vi "Final Project GUI with IMU.vi"() -> ()   [LabVIEW 2021]
doc: "This example performs writes and reads on a serial port, as directed by the user. You can press the Write and Read buttons, and change the Read Count, while the example is running.\n\nThe parameters set for the serial port must match the parameters of the connected instrument or device. In this example, the Read Count parameter specifies the number of bytes that the serial port reads. If there were more bytes at the port than the specified number, those bytes would not be read. If there were less bytes at the port than the specified number, you would receive a timeout error.\n\nThis example expands upon the flow control options for XON and XOFF, allowing the user to choose those control characters. Also, the user can enable or disable a termination character. Some devices require a termination character in order to identify the end of command strings. Some devices send a termination character to signify the end of data to be read. This example shows how you can end the Read operation once a termination character is detected in the buffer and/or append a termination character at the end of the Write data."
uses:
  Serial - Settings.ctl
  Serial - XON-XOFF Characters.ctl
  Serial - ASCII Characters-1.ctl
  <vilib>/Instr/_visa.llb/VISA Configure Serial Port (Instr).vi
  <vilib>/picture/picture.llb/Draw True-Color Pixmap.vi
panel:
  out "x*y":dbl
  out "front angle calcs":dbl
  out "ticks":dbl
  out "ResBack":dbl
  out "ResFront":dbl
  out "side angle calcs":dbl
  in  "milliseconds to wait":u32=17
  out "old pwm modifier":dbl
  in  "PWM actuator modifier":dbl
  out "Time used":dbl
  in  "Tab Control":T1(tab)
  in  "Write":bool
  out "Response":string
  in  "Command":string="\n\n"
  in  "Stop":bool
  in  "VISA resource name":refnum<visa-resource-name>="COM7"
  in  "Serial Settings":T2={"baud rate"=115200, "data bits"=8, "parity"=enum."None", "stop bits"=10, "flow control"=0} {"flow control" items=["None"=0, "XON/XOFF"=1, "RTS/CTS"=2, "DTR/DSR"=4]; "stop bits" items=["1.0"=10, "1.5"=15, "2.0"=20]; "data bits" min=5 max=8 step=1; "baud rate" items=["75"=75, "110"=110, "134"=134, "150"=150, "300"=300, "600"=600, "1200"=1200, "1800"=1800, "2400"=2400, "4800"=4800, "7200"=7200, "9600"=9600, "14400"=14400, "19200"=19200, "28800"=28800, "38400"=38400, "56000"=56000, "57600"=57600, "115200"=115200, "128000"=128000, "230400"=230400]}
  in  "End Read on Termination Character?":bool=TRUE
  in  "XON/XOFF Characters":T3={"XON"=enum."DC1", "XOFF"=enum."DC3"}
  in  "End Write on Termination Character?":bool=TRUE
  in  "Termination Character":u8=13 format="%.0x"
  out "Front View":picture
  out "Side View":picture
  out "Front View graph":dbl[](graph)
  out "Side Graph":dbl[](graph)
  in  "stop":bool
  out "IMU angle from PSOC":dbl
  in  "Reset Actuators to 2":bool
  in  "Reset Actuators to Zero":bool
  out "Actuator 1 Length (inches)":string
  out "Actuator 2 Length (inches)":string
  out "Actuator 3 Length (inches)":string
  out "Actuator 4 Length (inches)":string
  out "Actuator 1":dbl[](graph)
  out "Actuator 2":dbl[](graph)
  out "Actuator 3":dbl[](graph)
  out "Actuator 4":dbl[](graph)
  out "Actuator 1\nLength":dbl(slide) scale=0.0..2.0
  out "Actuator 2\nLength":dbl(slide) scale=0.0..2.0
  out "Actuator 3\nLength":dbl(slide) scale=0.0..2.0
  out "Actuator 4\nLength":dbl(slide) scale=0.0..2.0
  out "read buffer":string
  # "TEMPORARY DEBUGGING TOOLS"
  # "Hello! Welcome to the ME and the Boys ME135 Project!\n\nWe designed a mobile self-balancing platform with an actuator on each end. The rover will \nautomatically detect if the platform is not flat, and adjust the actuators accordingly while \ndriving over bumps and rough terrain.\n\nExplanation of each GUI tab:\nSetup - Serial Communication Setup (Change COM port here)\nOrientation Viewer - Plot of pitch and roll angle during operation \nActuator Lengths  - Plot of actuator lengths at each corner"
  # "Serial Communciation Setup Panel"
  # "Instructions:\n1. Using Windows Device Manager take note of the COM port given by Windows to your microcontroller connection\n2. Change the VISA resource name to your COM port from step 1\n3. Run the VI.\n4. Press reset on your microcontroller\n5. The corresponding response should appear in the Response Window\n6. Click Stop to stop the VI."
  # "0xA is equivalent to a '\\n' character, which is a line feed."
  # "Orientation\nViewer"
  # "Actuator Length Overview"
  # "CAR"
  # "car"
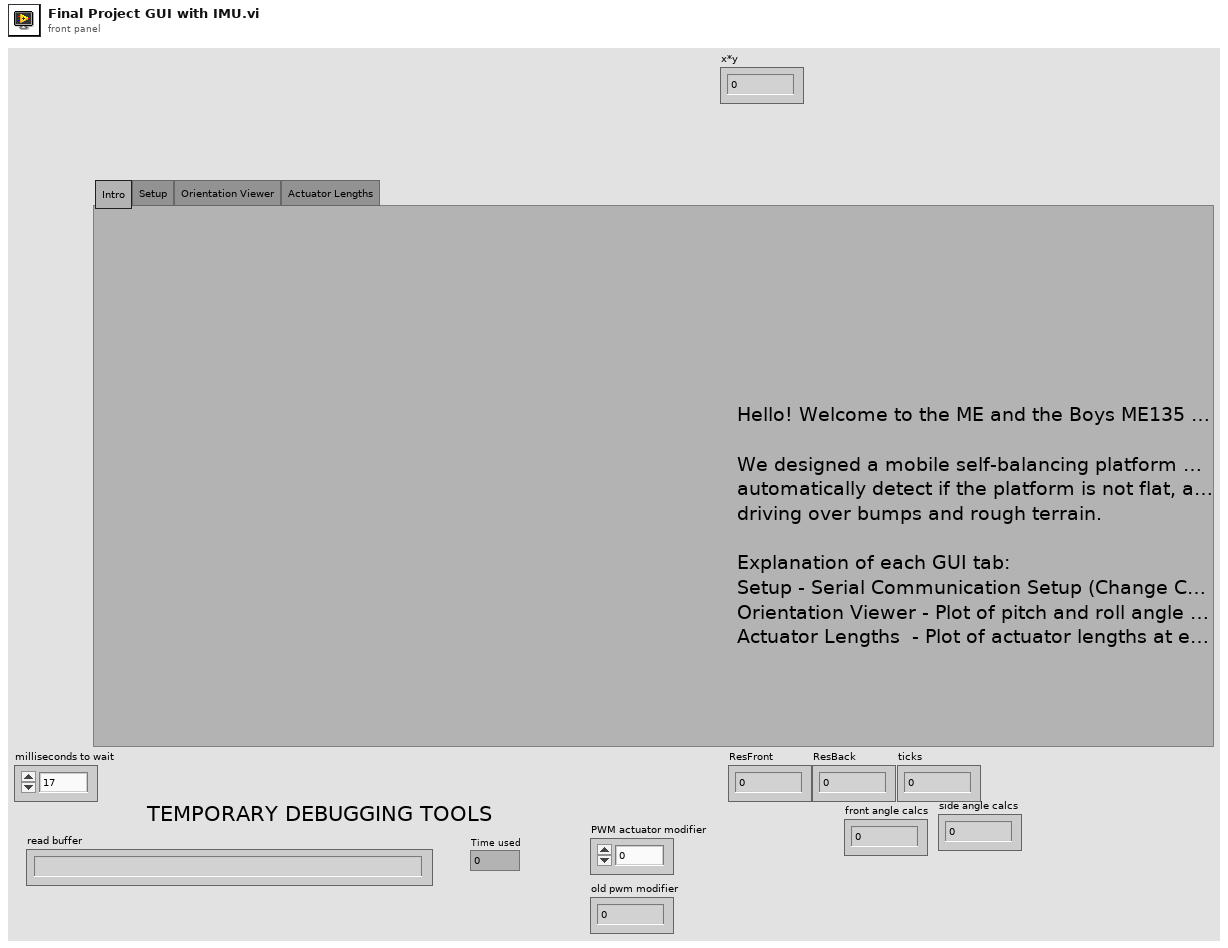
[diagram p1: front panel]
types:
  T1 = enum32{"Intro", "Setup", "Orientation Viewer", "Actuator Lengths"}
  T2 = typedef "Serial - Settings.ctl" = cluster{"baud rate":u32, "data bits":u16, "parity":enum16{"None", "Odd", "Even", "Mark", "Space"}, "stop bits":u16, "flow control":u16}
  T3 = typedef "Serial - XON-XOFF Characters.ctl" = cluster{"XON":T4, "XOFF":T4}
  T4 = typedef "Serial - ASCII Characters-1.ctl" = enum16{"NUL", "SOH", "STX", "ETX", "EOT", "ENQ", "ACK", "BEL", "BS", "HT", "LF", "VT", "FF", "CR", "SO", "SI", "DLE", "DC1", "DC2", "DC3", "DC4", "NAK", "SYN", "ETB", "CAN", "EM", "SUB", "ESC", "FS", "GS", "RS", "US", "SP", "!", "\"", "#", "$", "%", "&", "'", "(", ")", "*", "+", ",", "- (-)", ".", "/", "0", "1", "2", "3", "4", "5", "6", "7", "8", "9", ":", ";", "<", "=", ">", "?", "@", "A", "B", "C", "D", "E", "F", "G", "H", "I", "J", "K", "L", "M", "N", "O", "P", "Q", "R", "S", "T", "U", "V", "W", "X", "Y", "Z", "[", "\\", "]", "^", "_", "`", "a", "b", "c", "d", "e", "f", "g", "h", "i", "j", "k", "l", "m", "n", "o", "p", "q", "r", "s", "t", "u", "v", "w", "x", "y", "z", "{", "|", "}", "~"}
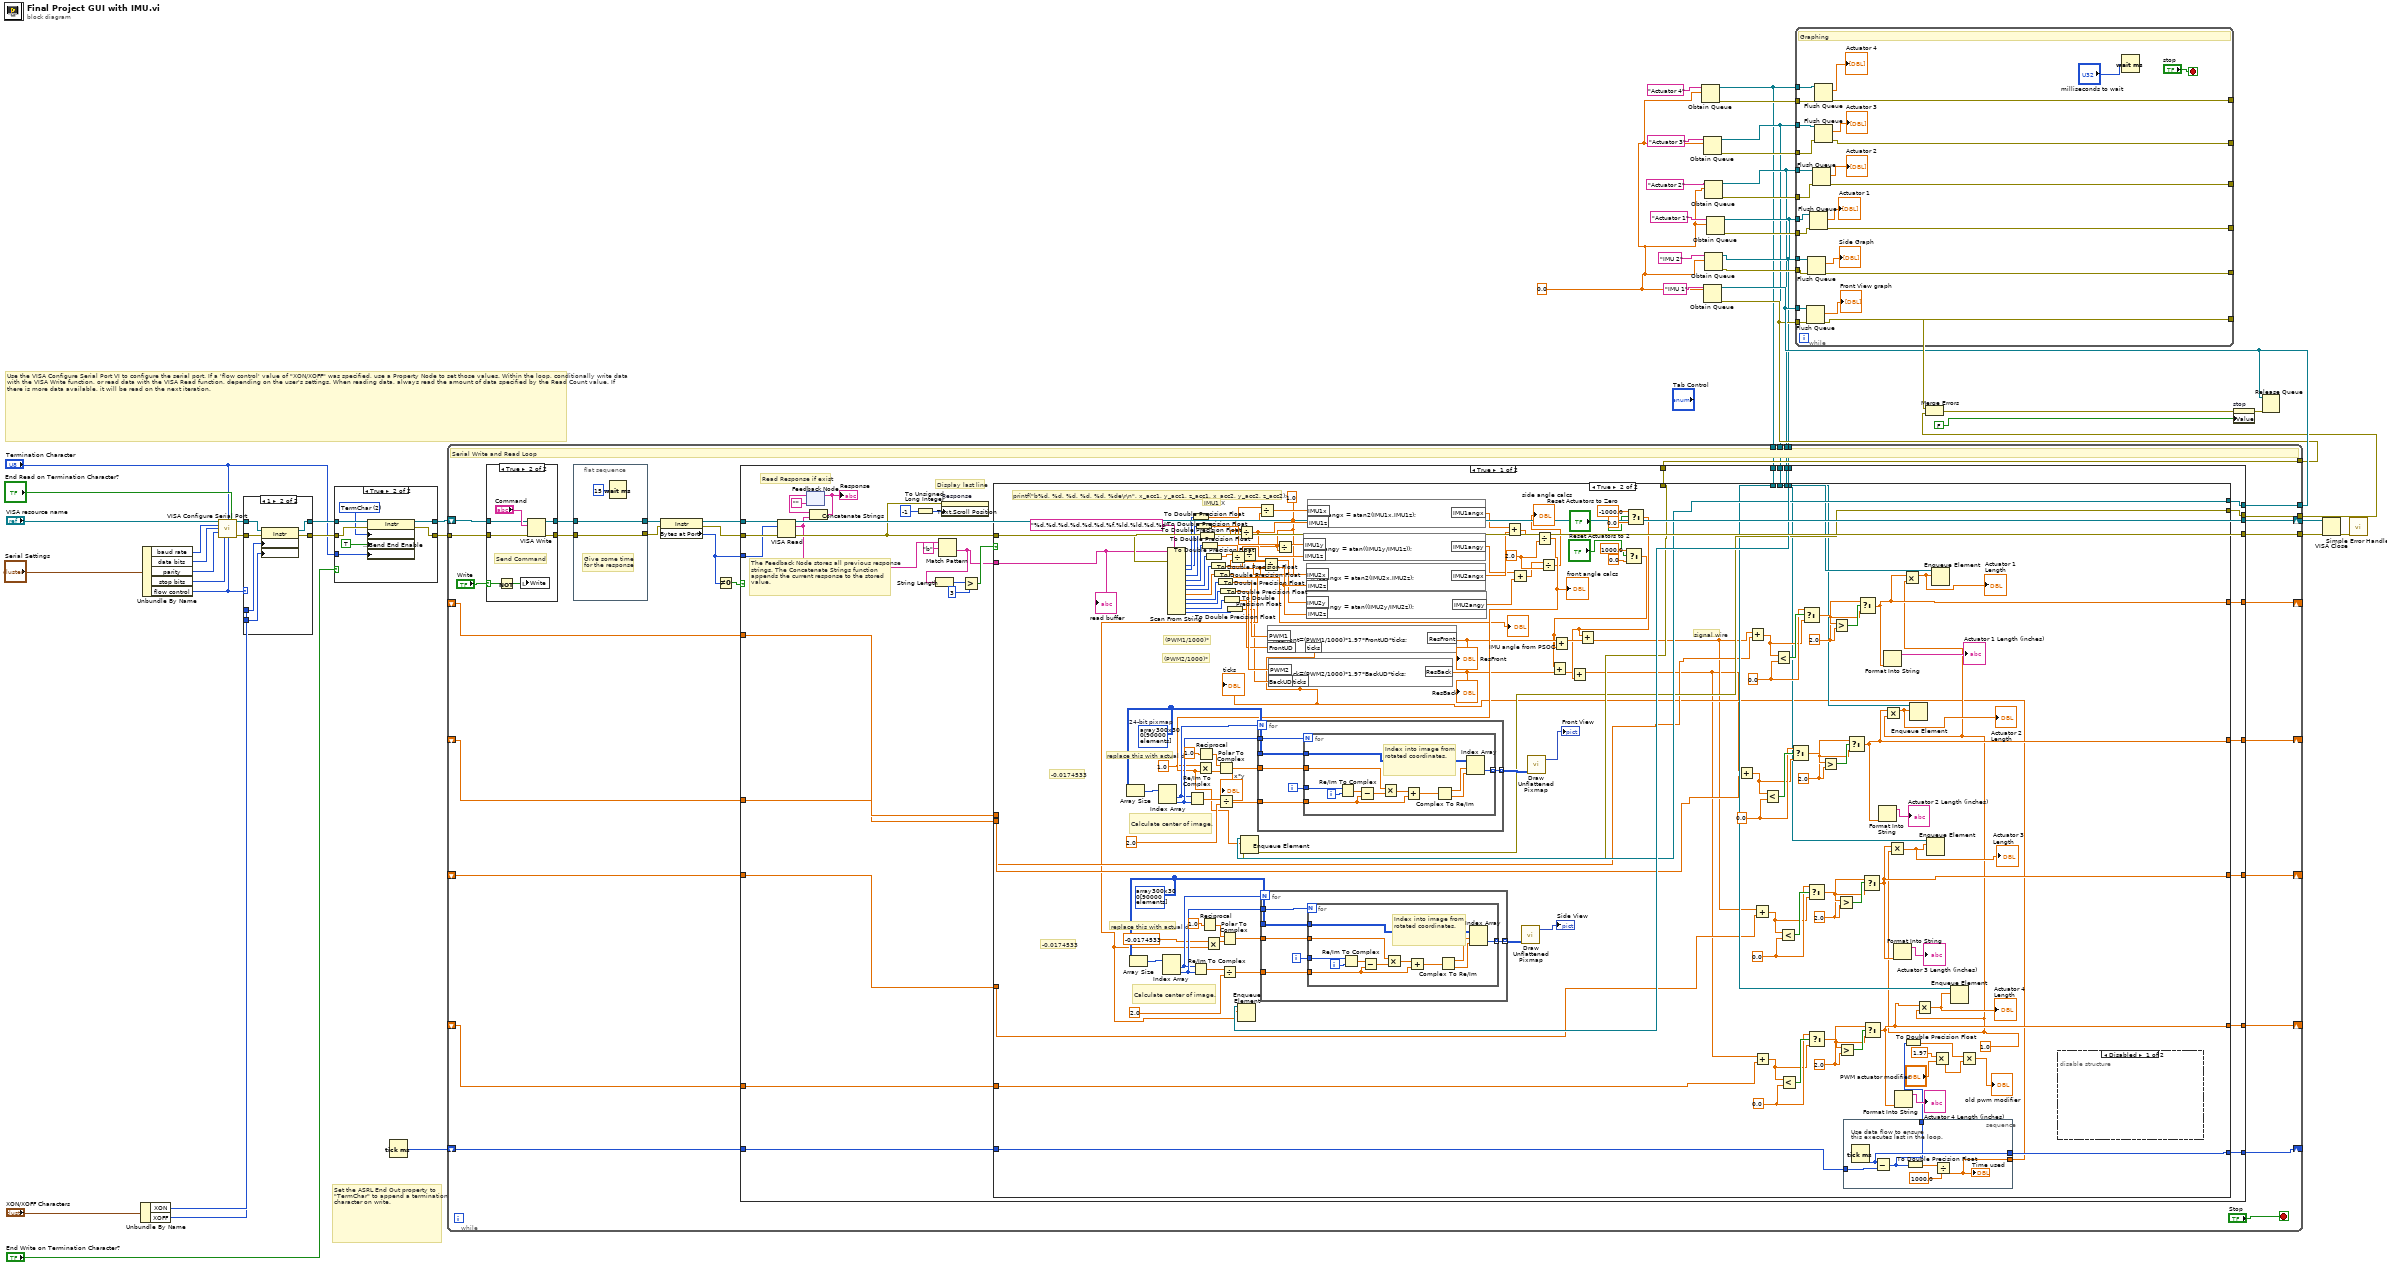
[diagram p0: block diagram]
diagram:
  w2 = 0.0
  # "Set the ASRL End Out property to \"TermChar\" to append a termination character on write."
  # "Use the VISA Configure Serial Port VI to configure the serial port. If a 'flow control' value of \"XON/XOFF\" was specified, use a Property Node to set those values. Within the loop, conditionally write data with the VISA Write function, or read data with the VISA Read function, depending on the user's settings. When reading data, always read the amount of data specified by the Read Count value. If there is more data available, it will be read on the next iteration."
  n1 = Unbundle By Name("XON/XOFF Characters") -> ("XON"=w33:T4, "XOFF"=w32:T4)
  n2 = Unbundle By Name("Serial Settings") -> ("baud rate"=w40:u32, "data bits"=w41:u16, "parity"=w42:enum16{"None", "Odd", "Even", "Mark", "Space"}, "stop bits"=w43:u16, "flow control"=w34:u16)
  n3 = call-poly "VISA Configure Serial Port"("VISA resource name"="VISA resource name", "termination char\n(0xA = '\\n' = LF)"="Termination Character", "Enable Termination\nChar (T)"="End Read on Termination Character?", "baud rate (9600)"=w40, "data bits (8)"=w41, "parity (0:none)"=w42, "stop bits (10: 1 bit)"=w43, "flow control (0:none)"=w34) -> ("VISA resource name out"=w44:refnum<visa-resource-name>, "error out"=w45:errorcluster)  [unwired: 2 in, 4 out]
  n4 = case shown="1" w34 {
    tunnel: [w48 w55] -> w31
    tunnel: [w49 w54] -> w29
    tunnel: w45 -> [w48 w53]
    tunnel: w44 -> [w49 w52]
    tunnel: w33 -> [_ w51]
    tunnel: w32 -> [_ w50]
    frame Default {
    }
    frame 1 {
      n5 = property class="Instr"(reference=w52, error in=w53, "Serial Settings:Flow Control XON Character"=w51, "Serial Settings:Flow Control XOFF Character"=w50) -> (reference out=w54:refnum<visa-resource-name>, error out=w55:errorcluster)
    }
  }
  n6 = case shown="True" "End Write on Termination Character?" {
    tunnel: w29 -> [w56 w64]
    tunnel: w31 -> [w57 w63]
    tunnel: [w56 w62] -> w28
    tunnel: [w57 w61] -> w30
    tunnel: "Termination Character" -> [_ w59]
    frame False {
    }
    frame True {
      w60 = u16 2 items=["None", "LastBit", "TermChar", "Break"] ("Serial Settings:Serial End Mode for Writes")
      n7 = property class="Instr"(reference=w64, error in=w63, "Serial Settings:End Mode for Writes"=w60, "Message Based Settings:Send End Enable"=TRUE, "Message Based Settings:Termination Character"=w59) -> (reference out=w62:refnum<visa-resource-name>, error out=w61:errorcluster)
    }
  }
  n8 = Tick Count (ms)() -> (millisecond timer value=w1:u32)
  n9 = Obtain Queue(name (unnamed)="Actuator 4", element data type=w2) -> (queue out=w3:refnum<queue>, error out=w13:errorcluster)  [unwired: 3 in, 1 out]
  n10 = Obtain Queue(name (unnamed)="Actuator 3", element data type=w2) -> (queue out=w4:refnum<queue>, error out=w14:errorcluster)  [unwired: 3 in, 1 out]
  n11 = Obtain Queue(name (unnamed)="IMU 1", element data type=w2) -> (queue out=w20:refnum<queue>, error out=w19:errorcluster)  [unwired: 3 in, 1 out]
  n12 = Obtain Queue(name (unnamed)="IMU 2", element data type=w2) -> (queue out=w7:refnum<queue>, error out=w17:errorcluster)  [unwired: 3 in, 1 out]
  n13 = Obtain Queue(name (unnamed)="Actuator 2", element data type=w2) -> (queue out=w5:refnum<queue>, error out=w15:errorcluster)  [unwired: 3 in, 1 out]
  n14 = Obtain Queue(name (unnamed)="Actuator 1", element data type=w2) -> (queue out=w6:refnum<queue>, error out=w16:errorcluster)  [unwired: 3 in, 1 out]
  n15 = while {
    shift-right: [w96] -> w35
    shift-left: w28 -> [w95]
    tunnel: w30 -> [w94]
    tunnel: [w93] -> w36
    tunnel: w20 -> [w83]
    tunnel: w19 -> [w82]
    tunnel: [w81] -> w18
    shift-right: [w80] -> _
    shift-left: _ -> [w79]
    shift-right: [w78] -> _
    shift-left: _ -> [w75]
    shift-right: [w77] -> _
    shift-left: _ -> [w74]
    shift-right: [w76] -> _
    shift-left: _ -> [w73]
    tunnel: w7 -> [w72]
    tunnel: w6 -> [w71]
    tunnel: w5 -> [w70]
    tunnel: w4 -> [w69]
    tunnel: w3 -> [w68]
    shift-right: [w67] -> _
    shift-left: w1 -> [w66]
    stop <- "Stop" stop-if-true
    # "Serial Write and Read Loop"
    n16 = case shown="True" "Write" {
      selector: "Write" -> [_ w103]
      tunnel: w95 -> [w101 w107]
      tunnel: w94 -> [w100 w106]
      tunnel: [w101 w105] -> w87
      tunnel: [w100 w104] -> w85
      frame False {
      }
      frame True {
        # "Send Command"
        n17 = Not(x=w103) -> (.not. x?=w102:bool)
        n18 = local write "Write"(w102) -> ()
        n19 = VISA Write(VISA resource name=w107, write buffer="Command", error in (no error)=w106) -> (VISA resource name out=w105:refnum<visa-resource-name>, error out=w104:errorcluster)  [unwired: 1 out]
      }
    }
    n20 = flat-sequence {
      tunnel: w87 -> [w99]
      tunnel: [w99] -> w86
      tunnel: w85 -> [w98]
      tunnel: [w98] -> w84
      frame #0 {
        # "Give some time\nfor the response"
        n21 = Wait (ms)(milliseconds to wait=u32 15) -> ()  [unwired: 1 out]
      }
    }
    n22 = property class="Instr"(reference=w86, error in=w84) -> (reference out=w90:refnum<visa-resource-name>, error out=w91:errorcluster, "Bytes at Port"=w88:u32)
    n23 = Not Equal To 0?(x=w88) -> (x != 0?=w89:bool)
    n24 = case shown="True" w89 {
      tunnel: [w136 w339] -> w96
      tunnel: w90 -> [w142 w339]
      tunnel: [w133 w338] -> w93
      tunnel: w91 -> [w141 w338]
      tunnel: w88 -> [w137 _]
      tunnel: w83 -> [w126 _]
      tunnel: w82 -> [w125 w337]
      tunnel: [w124 w337] -> w81
      tunnel: [w123 w336] -> w80
      tunnel: w79 -> [w122 w336]
      tunnel: [w121 w335] -> w78
      tunnel: [w120 w334] -> w77
      tunnel: [w119 w333] -> w76
      tunnel: w75 -> [w118 w335]
      tunnel: w74 -> [w117 w334]
      tunnel: w73 -> [w116 w333]
      tunnel: w72 -> [w115 _]
      tunnel: w71 -> [w114 _]
      tunnel: w70 -> [w113 _]
      tunnel: w69 -> [w112 _]
      tunnel: w68 -> [w111 _]
      tunnel: [w110 w332] -> w67
      tunnel: w66 -> [w109 w332]
      frame True {
        # "Read Response if exist"
        # "Display last line"
        # "The Feedback Node stores all previous response strings. The Concatenate Strings function appends the current response to the stored value."
        n25 = VISA Read(VISA resource name=w142, byte count=w137, error in (no error)=w141) -> (VISA resource name out=w136:refnum<visa-resource-name>, read buffer=w128:string, error out=w133:errorcluster)  [unwired: 1 out]
        n26 = feedback #1("") -> (w140:string)
        n27 = Concatenate Strings(w140, w128) -> (w139:string)
        "Response" <- w139
        n28 = feedback-in #1(w139) -> ()
        n29 = To Unsigned Long Integer(number=-1 ("Text.Scroll Position")) -> (unsigned 32bit integer=w134:u32)
        n30 = Match Pattern(string=w128, regular expression="b") -> (after substring=w127:string)  [unwired: 1 in, 3 out]
        n31 = String Length(string=w127) -> (length=w132:i32)
        n32 = property on="Response" class="Str"(error in=w133, "Text.Scroll Position"=w134) -> ()  [unwired: 1 in, 2 out]
        n33 = Greater?(x=w132, y=3) -> (0:w130:bool)
        n34 = case shown="True" w130 {
          tunnel: w133 -> [_ w289]
          tunnel: w127 -> [_ w287]
          tunnel: w126 -> [_ w230]
          tunnel: w125 -> [w144 w229]
          tunnel: [w144 w228] -> w124
          tunnel: [w146 w227] -> w123
          tunnel: w122 -> [w146 w217]
          tunnel: [w145 w225] -> w121
          tunnel: [w147 w223] -> w120
          tunnel: [w148 w194] -> w119
          tunnel: w118 -> [w145 w218]
          tunnel: w117 -> [w147 w219]
          tunnel: w116 -> [w148 w220]
          tunnel: w115 -> [_ w231]
          tunnel: w114 -> [_ w226]
          tunnel: w113 -> [_ w224]
          tunnel: w112 -> [_ w222]
          tunnel: w111 -> [_ w221]
          tunnel: [w143 w195] -> w110
          tunnel: w109 -> [w143 w196]
          frame False {
          }
          frame True {
            w149 = 1.0 ("y")
            w184 = 1.0 ("y")
            w200 = 2.0
            w232 = u32[][] array300x300[90000 elements] ("24-bit pixmap")
            w238 = 0.0
            w234 = 2.0
            w245 = 0.0
            w241 = 2.0
            w252 = 0.0
            w248 = 2.0
            w259 = 0.0
            w255 = 2.0
            w273 = u32[][] array300x300[90000 elements]  # 24-bit pixmap
            # "-0.0174533"
            # "-0.0174533"
            # "(PWM1/1000)*"
            # "(PWM2/1000)*"
            # "printf(\"b%d, %d, %d, %d, %d, %de\\r\\n\", x_acc1, y_acc1, z_acc1, x_acc2, y_acc2, z_acc2);"
            # "IMU1 X"
            # "signal wire"
            # "replace this with actual data"
            # "Calculate center of image."
            # "replace this with actual data"
            # "Calculate center of image."
            n35 = Array Size(array=w273) -> (size(s)=w279:i32[])
            n36 = Array Size(array=w232) -> (size(s)=w267:i32[])
            n37 = Index Array(array=w279) -> (element #1=w277:i32, element #2=w278:i32)  [unwired: 2 in]
            n38 = Index Array(array=w267) -> (element #1=w265:i32, element #2=w266:i32)  [unwired: 2 in]
            n39 = Scan From String(format string="%d,%d,%d,%d,%d,%d,%f,%ld,%ld,%d,%d", input string=w287, error in=w289) -> (output 1=w286:i32, output 2=w285:i32, output 3=w216:i32, output 4=w215:i32, output 5=w214:i32, output 6=w213:i32, output 7=w212:dbl, output 8=w211:i32, output 9=w210:i32, output 10=w209:i32, output 11=w208:i32)  [unwired: 12 in, 3 out]
            n40 = Re/Im To Complex(1:w278, 2:w277) -> (0:w280:cdb)
            n41 = To Double Precision Float(number=w286) -> (double precision float=w284:dbl)
            n42 = Re/Im To Complex(1:w266, 2:w265) -> (0:w268:cdb)
            n43 = To Double Precision Float(number=w285) -> (double precision float=w207:dbl)
            n44 = Reciprocal(x=1.0) -> (1/x=w281:dbl)
            n45 = To Double Precision Float(number=w216) -> (double precision float=w154:dbl)
            n46 = Reciprocal(x=1.0) -> (1/x=w269:dbl)
            n47 = To Double Precision Float(number=w215) -> (double precision float=w151:dbl)
            n48 = To Double Precision Float(number=w214) -> (double precision float=w205:dbl)
            n49 = To Double Precision Float(number=w213) -> (double precision float=w206:dbl)
            n50 = To Double Precision Float(number=w212) -> (double precision float=w178:dbl)
            "IMU angle from PSOC" <- w178
            n51 = Multiply(x=-0.0174533, y=w178) -> (x*y=w176:dbl)
            n52 = To Double Precision Float(number=w211) -> (double precision float=w183:dbl)
            n53 = Divide(x=w280, y=2.0) -> (x/y=w276:cdb)
            n54 = To Double Precision Float(number=w210) -> (double precision float=w182:dbl)
            n55 = Polar To Complex(1:w176, 2:w269) -> (0:w262:cdb)
            n56 = Divide(x=w268, y=2.0) -> (x/y=w264:cdb)
            n57 = To Double Precision Float(number=w209) -> (double precision float=w181:dbl)
            n58 = To Double Precision Float(number=w208) -> (double precision float=w172:dbl)
            n59 = Divide(x=w205, y=w149) -> (x/y=w150:dbl)
            n60 = Enqueue Element(queue=w231, element=w178) -> ()  [unwired: 2 in, 3 out]
            n61 = Divide(x=w154, y=w149) -> (x/y=w155:dbl)
            n62 = Divide(x=w151, y=w149) -> (x/y=w152:dbl)
            n63 = Divide(x=w284, y=w149) -> (x/y=w157:dbl)
            n64 = for {
              N: w265 -> [_]
              tunnel: w266 -> [w300]
              tunnel: w232 -> [w299]
              tunnel: [w298] -> w271 mode=indexing
              tunnel: w262 -> [w297]
              tunnel: w264 -> [w296]
              i -> [w301]
              n65 = for {
                N: w300 -> [_]
                tunnel: w301 -> [w310]
                tunnel: w299 -> [w313]
                tunnel: [w312] -> w298 mode=indexing
                tunnel: w297 -> [w307]
                tunnel: w296 -> [w302]
                i -> [w311]
                # "Index into image from rotated coordinates."
                n66 = Re/Im To Complex(1:w311, 2:w310) -> (0:w309:cdb)
                n67 = Subtract(x=w309, y=w302) -> (x-y=w308:cdb)
                n68 = Multiply(x=w307, y=w308) -> (x*y=w306:cdb)
                n69 = Add(x=w306, y=w302) -> (x+y=w305:cdb)
                n70 = Complex To Re/Im(x + iy=w305) -> (x=w304:dbl, y=w303:dbl)
                n71 = Index Array(array=w313, index (row)=w304, index (col)=w303) -> (element=w312:u32)
              }
            }
            n72 = Divide(x=w206, y=w149) -> (x/y=w153:dbl)
            n73 = Divide(x=w207, y=w149) -> (x/y=w156:dbl)
            n74 = formula code="IMU1angy = atan((IMU1y/IMU1z));"("IMU1y"=w156, "IMU1z"=w155) -> ("IMU1angy"=w202:dbl)
            n75 = formula code="IMU2angx = atan2(IMU2x,IMU2z);"("IMU2x"=w152, "IMU2z"=w153) -> ("IMU2angx"=w203:dbl)
            n76 = formula code="IMU2angy = atan((IMU2y/IMU2z));"("IMU2y"=w150, "IMU2z"=w153) -> ("IMU2angy"=w201:dbl)
            n77 = formula code="IMU1angx = atan2(IMU1x,IMU1z);"("IMU1x"=w157, "IMU1z"=w155) -> ("IMU1angx"=w204:dbl)
            n78 = Add(x=w204, y=w203) -> (x+y=w199:dbl)
            n79 = Add(x=w202, y=w201) -> (x+y=w198:dbl)
            n80 = call-poly <vilib>:"Draw Unflattened Pixmap.vi"("data (RGB format)"=w271) -> ("new picture"=→"Side View":picture)  [unwired: 8 in]
            n81 = Divide(x=w199, y=w200) -> (x/y=w197:dbl)
            "front angle calcs" <- w197
            n82 = Multiply(x=1.0, y=w197) -> (x*y=w174:dbl)
            "x*y" <- w174
            n83 = Polar To Complex(1:w174, 2:w281) -> (0:w274:cdb)
            n84 = Enqueue Element(queue=w230, element=w197, error in (no error)=w229) -> (error out=w228:errorcluster)  [unwired: 1 in, 2 out]
            n85 = for {
              N: w277 -> [_]
              tunnel: w278 -> [w318]
              tunnel: w273 -> [w317]
              tunnel: [w316] -> w283 mode=indexing
              tunnel: w274 -> [w315]
              tunnel: w276 -> [w314]
              i -> [w319]
              n86 = for {
                N: w318 -> [_]
                tunnel: w319 -> [w328]
                tunnel: w317 -> [w331]
                tunnel: [w330] -> w316 mode=indexing
                tunnel: w315 -> [w325]
                tunnel: w314 -> [w320]
                i -> [w329]
                # "Index into image from rotated coordinates."
                n87 = Re/Im To Complex(1:w329, 2:w328) -> (0:w327:cdb)
                n88 = Subtract(x=w327, y=w320) -> (x-y=w326:cdb)
                n89 = Multiply(x=w325, y=w326) -> (x*y=w324:cdb)
                n90 = Add(x=w324, y=w320) -> (x+y=w323:cdb)
                n91 = Complex To Re/Im(x + iy=w323) -> (x=w322:dbl, y=w321:dbl)
                n92 = Index Array(array=w331, index (row)=w322, index (col)=w321) -> (element=w330:u32)
              }
            }
            n93 = call-poly <vilib>:"Draw Unflattened Pixmap.vi"("data (RGB format)"=w283) -> ("new picture"=→"Front View":picture)  [unwired: 8 in]
            n94 = Divide(x=w198, y=w200) -> (x/y=→"side angle calcs":dbl)
            n95 = Select(t=1000.0, s="Reset Actuators to 2", f=0.0) -> (s? t:f=w158:dbl)
            n96 = Select(t=-1000.0, s="Reset Actuators to Zero", f=0.0) -> (s? t:f=w160:dbl)
            n97 = stacked-sequence {
              tunnel: w196 -> [w295]
              tunnel: [w294] -> w195
              tunnel: [w292] -> w193
              tunnel: [w290] -> w170
              frame #0 {
                # "Use data flow to ensure\nthis executes last in the loop."
                n98 = Tick Count (ms)() -> (millisecond timer value=w294:u32)
                n99 = Subtract(x=w294, y=w295) -> (x-y=w292:u32)
                n100 = To Double Precision Float(number=w292) -> (double precision float=w291:dbl)
                n101 = Divide(x=w291, y=1000.0) -> (x/y=w290:dbl)
                "Time used" <- w290
              }
            }
            "ticks" <- w170
            n102 = formula code="ResFront=(PWM1/1000)*1.97*FrontUD*ticks;"("PWM1"=w183, "FrontUD"=w181, "ticks"=w170) -> ("ResFront"=w180:dbl)
            "ResFront" <- w180
            n103 = formula code="ResBack=(PWM2/1000)*1.97*BackUD*ticks;"("PWM2"=w182, "BackUD"=w172, "ticks"=w170) -> ("ResBack"=w179:dbl)
            "ResBack" <- w179
            n104 = Add(x=w158, y=w179) -> (x+y=w159:dbl)
            n105 = Add(x=w180, y=w158) -> (x+y=w161:dbl)
            n106 = Add(x=w159, y=w160) -> (x+y=w162:dbl)
            n107 = Add(x=w160, y=w161) -> (x+y=w163:dbl)
            n108 = Add(x=w162, y=w218) -> (x+y=w251:dbl)
            n109 = Add(x=w163, y=w217) -> (x+y=w258:dbl)
            n110 = Add(x=w163, y=w219) -> (x+y=w244:dbl)
            n111 = Add(x=w162, y=w220) -> (x+y=w237:dbl)
            n112 = Less?(x=w251, y=w252) -> (x < y?=w253:bool)
            n113 = Less?(x=w258, y=w259) -> (x < y?=w260:bool)
            n114 = Less?(x=w244, y=w245) -> (x < y?=w246:bool)
            n115 = Less?(x=w237, y=w238) -> (x < y?=w239:bool)
            n116 = Select(t=w252, s=w253, f=w251) -> (s? t:f=w249:dbl)
            n117 = Select(t=w259, s=w260, f=w258) -> (s? t:f=w256:dbl)
            n118 = Select(t=w245, s=w246, f=w244) -> (s? t:f=w242:dbl)
            n119 = Select(t=w238, s=w239, f=w237) -> (s? t:f=w235:dbl)
            n120 = Greater?(x=w249, y=w248) -> (0:w250:bool)
            n121 = Greater?(x=w256, y=w255) -> (0:w257:bool)
            n122 = Greater?(x=w242, y=w241) -> (0:w243:bool)
            n123 = Greater?(x=w235, y=w234) -> (0:w236:bool)
            n124 = Select(t=w248, s=w250, f=w249) -> (s? t:f=w225:dbl)
            n125 = Select(t=w255, s=w257, f=w256) -> (s? t:f=w227:dbl)
            n126 = Select(t=w241, s=w243, f=w242) -> (s? t:f=w223:dbl)
            n127 = Select(t=w234, s=w236, f=w235) -> (s? t:f=w194:dbl)
            n128 = Format Into String(w225) -> (resulting string=→"Actuator 2 Length (inches)":string)  [unwired: 3 in, 1 out]
            n129 = Format Into String(w227) -> (resulting string=→"Actuator 1 Length (inches)":string)  [unwired: 3 in, 1 out]
            n130 = Multiply(x=w225, y=w184) -> (x*y=w188:dbl)
            "Actuator 2\nLength" <- w188
            n131 = Multiply(x=w223, y=w184) -> (x*y=w189:dbl)
            "Actuator 3\nLength" <- w189
            n132 = Format Into String(w223) -> (resulting string=→"Actuator 3 Length (inches)":string)  [unwired: 3 in, 1 out]
            n133 = Format Into String(w194) -> (resulting string=→"Actuator 4 Length (inches)":string)  [unwired: 3 in, 1 out]
            n134 = Multiply(x=w227, y=w184) -> (x*y=w187:dbl)
            "Actuator 1\nLength" <- w187
            n135 = To Double Precision Float(number=w193) -> (double precision float=w192:dbl)
            n136 = Enqueue Element(queue=w224, element=w188) -> ()  [unwired: 2 in, 3 out]
            n137 = Multiply(x=w194, y=w184) -> (x*y=w190:dbl)
            "Actuator 4\nLength" <- w190
            n138 = Enqueue Element(queue=w222, element=w189) -> ()  [unwired: 2 in, 3 out]
            n139 = Enqueue Element(queue=w226, element=w187) -> ()  [unwired: 2 in, 3 out]
            n140 = Multiply(x=1.97, y="PWM actuator modifier") -> (x*y=w186:dbl)
            n141 = Enqueue Element(queue=w221, element=w190) -> ()  [unwired: 2 in, 3 out]
            n142 = Multiply(x=w192, y=w186) -> (x*y=→"old pwm modifier":dbl)
            n143 = disable-structure shown="Disabled" {
              frame Disabled {
              }
              frame Enabled {
              }
            }
            "read buffer" <- w287
          }
        }
      }
      frame False {
      }
    }
  }
  n144 = while {
    tunnel: w20 -> [w365]
    tunnel: w19 -> [w363]
    tunnel: [w362] -> w24
    tunnel: w3 -> [w359]
    tunnel: w4 -> [w358]
    tunnel: w5 -> [w357]
    tunnel: w6 -> [w356]
    tunnel: w7 -> [w355]
    tunnel: [w354] -> _
    tunnel: w17 -> [w353]
    tunnel: w16 -> [w352]
    tunnel: [w351] -> _
    tunnel: w15 -> [w350]
    tunnel: [w349] -> _
    tunnel: w14 -> [w345]
    tunnel: [w344] -> _
    tunnel: w13 -> [w343]
    tunnel: [w342] -> _
    stop <- "stop" stop-if-true
    # "Graphing"
    n145 = Flush Queue(queue=w365, error in (no error)=w363) -> (remaining elements=→"Front View graph":dbl[], error out=w362:errorcluster)  [unwired: 1 out]
    n146 = Flush Queue(queue=w355, error in (no error)=w353) -> (remaining elements=→"Side Graph":dbl[], error out=w354:errorcluster)  [unwired: 1 out]
    n147 = Flush Queue(queue=w356, error in (no error)=w352) -> (remaining elements=→"Actuator 1":dbl[], error out=w351:errorcluster)  [unwired: 1 out]
    n148 = Flush Queue(queue=w357, error in (no error)=w350) -> (remaining elements=→"Actuator 2":dbl[], error out=w349:errorcluster)  [unwired: 1 out]
    n149 = Flush Queue(queue=w359, error in (no error)=w343) -> (remaining elements=→"Actuator 4":dbl[], error out=w342:errorcluster)  [unwired: 1 out]
    n150 = Flush Queue(queue=w358, error in (no error)=w345) -> (remaining elements=→"Actuator 3":dbl[], error out=w344:errorcluster)  [unwired: 1 out]
    n151 = Wait (ms)(milliseconds to wait="milliseconds to wait") -> ()  [unwired: 1 out]
  }
  n152 = Merge Errors(w24, w18) -> (w23:errorcluster)
  n153 = property on="stop" class="Bool (strict)"(error in=w23, "Value"=FALSE ("stop")) -> (error out=w22:errorcluster)  [unwired: 1 in, 1 out]
  n154 = Release Queue(queue=w20, error in (no error)=w22) -> ()  [unwired: 1 in, 3 out]
  n155 = VISA Close(VISA resource name=w35, error in (no error)=w36) -> (error out=w37:errorcluster)
  n156 = call <vilib>:"Simple Error Handler.vi"("error in (no error)"=w37) -> ()  [unwired: 1 in, 8 out]
